vi "MultipleMissions.vi"   [LabVIEW 2014, in "LegoMindstormProjects.lvrbt"]
uses:
  LegoMindstormProjects.lvrbt
  <vilib>/NXT/Block Support/NXT_InputPort.ctl
  <vilib>/NXT/Block Support/NXT_OutputPort.ctl
  <vilib>/NXT/Subs/ColorSensorColors.ctl
  <vilib>/NXT/Dual Mode Library/Sensors/EV3_Gyro_Reset.vi
  <vilib>/NXT/NXTIO Xnodes/NXTIONodeSubVIs/NXTMoveMotors.vi
  <vilib>/NXT/Dual Mode Library/Waits/Wait_Num.vi
  <vilib>/NXT/Dual Mode Library/Sensors/EV3_Color_Color.vi
  <vilib>/NXT/NXTIO Xnodes/NXTIONodeSubVIs/NXTStopMotors.vi
  <vilib>/NXT/Dual Mode Library/Waits/Wait_EV3_Angle_Greater.vi
  <vilib>/NXT/Dual Mode Library/Waits/Wait_Rotation.vi
  <vilib>/NXT/Dual Mode Library/Waits/Wait_EV3_Angle_Less.vi
  <vilib>/NXT/NXTIO Xnodes/AddressXNode/NXTIOAddress.xnode
  <vilib>/NXT/NXTIO Xnodes/NXTIOXNode/NXTIO.xnode
  <vilib>/NXT/Subs/LVHSConnector.ctl
  <vilib>/NXT/LegoClasses/BrickReference/BrickReference.lvclass
types:
  T1 = typedef "NXT_InputPort.ctl" = u32
  T2 = typedef "NXT_OutputPort.ctl" = u8
  T3 = typedef "LVHSConnector.ctl" = refnum<class "BrickReference.lvclass">
  T4 = typedef "ColorSensorColors.ctl" = enum16{"No Color", "Black", "Blue", "Green", "Yellow", "Red", "White", "Brown"}
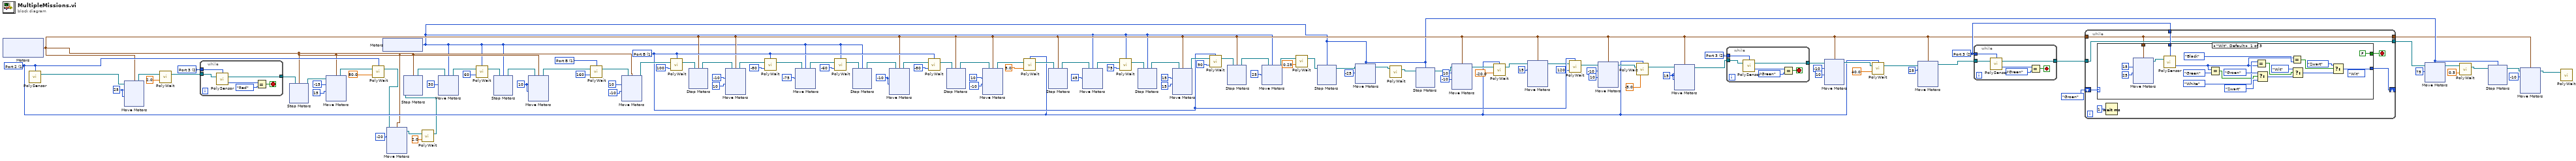
[diagram p0: block diagram]
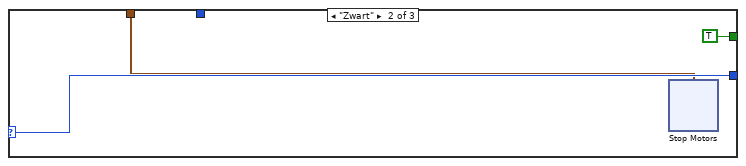
[diagram p2: hidden frame]
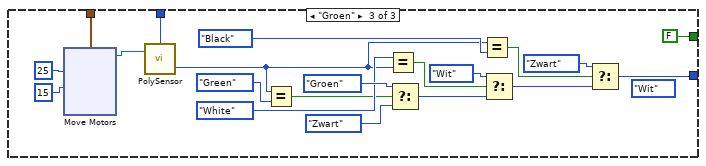
[diagram p3: hidden frame]
diagram:
  w2 = i8 -10 ("Power/Speed 1")
  w15 = i8 -20 ("Power/Speed 1")
  w19 = T1 2 items=["Port 1", "Port 2", "Port 3", "Port 4"] ("Port (Port 1)")
  w23 = i8 25 ("Power/Speed 1")
  w32 = i8 15 ("Power/Speed 1")
  w36 = T1 2 items=["Port 1", "Port 2", "Port 3", "Port 4"] ("Port (Port 1)")
  w42 = i8 15 ("Power/Speed 1")
  w59 = i8 25 ("Power/Speed 1")
  w82 = i8 -10 ("Power/Speed 1")
  w41 = T2 1 items=["Port A", "Port B", "Port C", "Port D"] ("Port (Port A)")
  w101 = T2 1 items=["Port A", "Port B", "Port C", "Port D"] ("Port (Port A)")
  w103 = i8 10 ("Power/Speed 2")
  w26 = T1 1 items=["Port 1", "Port 2", "Port 3", "Port 4"] ("Port (Port 1)")
  w116 = T1 2 items=["Port 1", "Port 2", "Port 3", "Port 4"] ("Port (Port 1)")
  n1 = xnode "Motors"() -> ("Motor"=w17:cluster{"Port":T2, "Port":T2})
  n2 = call-poly <vilib>:"PolySensor.vi"("Port (Port 1)"=w26) -> ("NXT/EV3"=w11:T3)  [unwired: 3 in]
  n3 = xnode "Move Motors"("Power/Speed 2"=w59, "Power/Speed 1"=w59, "Motors"=w17, "NXT/EV3"=w11) -> ("NXT/EV3"=w57:T3)
  n4 = call-poly <vilib>:"PolyWait.vi"("Time (1 sec)"=sgl 2.0, "NXT/EV3"=w57) -> ("NXT/EV3"=w56:T3)  [unwired: 2 in]
  n5 = while {
    tunnel: w116 -> [w122]
    tunnel: [w118] -> w115
    tunnel: w56 -> [w117]
    stop <- w119 stop-if-true
    n6 = call-poly <vilib>:"PolySensor.vi"("NXT/EV3"=w117, "Port (Port 1)"=w122) -> ("Detected Color"=w121:T4, "NXT/EV3"=w118:T3)  [unwired: 1 in]
    n7 = Equal?(x=w121, y=ColorSensorColors."Red") -> (x = y?=w119:bool)
  }
  n8 = xnode "Stop Motors"("Motors"=w17, "NXT/EV3"=w115) -> ("NXT/EV3"=w114:T3)
  n9 = xnode "Move Motors"("Power/Speed 2"=i8 15, "Power/Speed 1"=i8 -15, "Motors"=w17, "NXT/EV3"=w114) -> ("NXT/EV3"=w110:T3)
  n10 = call-poly <vilib>:"PolyWait.vi"("Degrees (180)"=sgl 80.0, "NXT/EV3"=w110, "Port (Port 1)"=w26) -> ("NXT/EV3"=w16:T3)  [unwired: 1 in]
  n11 = xnode "Motors"() -> ("Motor"=w5:T2)
  n12 = xnode "Move Motors"("Power/Speed 2"=w15, "Power/Speed 1"=w15, "Motors"=w17, "NXT/EV3"=w16) -> ("NXT/EV3"=w14:T3)
  n13 = call-poly <vilib>:"PolyWait.vi"("Time (1 sec)"=sgl 2.0, "NXT/EV3"=w14) -> ("NXT/EV3"=w12:T3)  [unwired: 2 in]
  n14 = xnode "Stop Motors"("Motors"=w17, "NXT/EV3"=w12) -> ("NXT/EV3"=w109:T3)
  n15 = xnode "Move Motors"("Power/Speed 1"=i8 30, "Motors"=w5, "NXT/EV3"=w109) -> ("NXT/EV3"=w107:T3)
  n16 = call-poly <vilib>:"PolyWait.vi"("Position Change (180)"=60, "NXT/EV3"=w107, "Port (Port A)"=w5) -> ("NXT/EV3"=w105:T3)  [unwired: 1 in]
  n17 = xnode "Stop Motors"("Motors"=w5, "NXT/EV3"=w105) -> ("NXT/EV3"=w104:T3)
  n18 = xnode "Move Motors"("Power/Speed 2"=w103, "Power/Speed 1"=w103, "Motors"=w17, "NXT/EV3"=w104) -> ("NXT/EV3"=w102:T3)
  n19 = call-poly <vilib>:"PolyWait.vi"("Position Change (180)"=160, "NXT/EV3"=w102, "Port (Port A)"=w101) -> ("NXT/EV3"=w99:T3)  [unwired: 1 in]
  n20 = xnode "Move Motors"("Power/Speed 2"=i8 -10 ("Power/Speed 1"), "Power/Speed 1"=i8 10, "Motors"=w17, "NXT/EV3"=w99) -> ("NXT/EV3"=w97:T3)
  n21 = call-poly <vilib>:"PolyWait.vi"("Position Change (180)"=100, "NXT/EV3"=w97, "Port (Port A)"=w41) -> ("NXT/EV3"=w96:T3)  [unwired: 1 in]
  n22 = xnode "Stop Motors"("Motors"=w17, "NXT/EV3"=w96) -> ("NXT/EV3"=w95:T3)
  n23 = xnode "Move Motors"("Power/Speed 2"=i8 10 ("Power/Speed 1"), "Power/Speed 1"=i8 -10, "Motors"=w17, "NXT/EV3"=w95) -> ("NXT/EV3"=w94:T3)
  n24 = call-poly <vilib>:"PolyWait.vi"("Position Change (180)"=-80, "NXT/EV3"=w94, "Port (Port A)"=w41) -> ("NXT/EV3"=w86:T3)  [unwired: 1 in]
  n25 = xnode "Move Motors"("Power/Speed 1"=i8 -75, "Motors"=w5, "NXT/EV3"=w86) -> ("NXT/EV3"=w84:T3)
  n26 = call-poly <vilib>:"PolyWait.vi"("Position Change (180)"=-60, "NXT/EV3"=w84, "Port (Port A)"=w5) -> ("NXT/EV3"=w74:T3)  [unwired: 1 in]
  n27 = xnode "Stop Motors"("Motors"=w5, "NXT/EV3"=w74) -> ("NXT/EV3"=w73:T3)
  n28 = xnode "Move Motors"("Power/Speed 2"=w82, "Power/Speed 1"=w82, "Motors"=w17, "NXT/EV3"=w73) -> ("NXT/EV3"=w88:T3)
  n29 = call-poly <vilib>:"PolyWait.vi"("Position Change (180)"=-80, "NXT/EV3"=w88, "Port (Port A)"=w41) -> ("NXT/EV3"=w81:T3)  [unwired: 1 in]
  n30 = xnode "Stop Motors"("Motors"=w17, "NXT/EV3"=w81) -> ("NXT/EV3"=w80:T3)
  n31 = xnode "Move Motors"("Power/Speed 2"=i8 -10, "Power/Speed 1"=i8 10, "Motors"=w17, "NXT/EV3"=w80) -> ("NXT/EV3"=w77:T3)
  n32 = call-poly <vilib>:"PolyWait.vi"("Degrees (180)"=sgl 5.0, "NXT/EV3"=w77, "Port (Port 1)"=w26) -> ("NXT/EV3"=w76:T3)  [unwired: 1 in]
  n33 = xnode "Stop Motors"("Motors"=w17, "NXT/EV3"=w76) -> ("NXT/EV3"=w72:T3)
  n34 = xnode "Move Motors"("Power/Speed 1"=i8 45, "Motors"=w5, "NXT/EV3"=w72) -> ("NXT/EV3"=w70:T3)
  n35 = call-poly <vilib>:"PolyWait.vi"("Position Change (180)"=75, "NXT/EV3"=w70, "Port (Port A)"=w5) -> ("NXT/EV3"=w67:T3)  [unwired: 1 in]
  n36 = xnode "Stop Motors"("Motors"=w5, "NXT/EV3"=w67) -> ("NXT/EV3"=w68:T3)
  n37 = xnode "Move Motors"("Power/Speed 2"=i8 15, "Power/Speed 1"=i8 15, "Motors"=w17, "NXT/EV3"=w68) -> ("NXT/EV3"=w64:T3)
  n38 = call-poly <vilib>:"PolyWait.vi"("Position Change (180)"=90, "NXT/EV3"=w64, "Port (Port A)"=w41) -> ("NXT/EV3"=w62:T3)  [unwired: 1 in]
  n39 = xnode "Stop Motors"("Motors"=w17, "NXT/EV3"=w62) -> ("NXT/EV3"=w61:T3)
  n40 = xnode "Move Motors"("Power/Speed 1"=i8 25, "Motors"=w5, "NXT/EV3"=w61) -> ("NXT/EV3"=w54:T3)
  n41 = call-poly <vilib>:"PolyWait.vi"("Time (1 sec)"=sgl 0.25, "NXT/EV3"=w54) -> ("NXT/EV3"=w55:T3)  [unwired: 2 in]
  n42 = xnode "Stop Motors"("Motors"=w5, "NXT/EV3"=w55) -> ("NXT/EV3"=w50:T3)
  n43 = xnode "Move Motors"("Power/Speed 1"=i8 -25, "Motors"=w5, "NXT/EV3"=w50) -> ("NXT/EV3"=w52:T3)
  n44 = call-poly <vilib>:"PolyWait.vi"("NXT/EV3"=w52) -> ("NXT/EV3"=w51:T3)  [unwired: 3 in]
  n45 = xnode "Stop Motors"("Motors"=w5, "NXT/EV3"=w51) -> ("NXT/EV3"=w48:T3)
  n46 = xnode "Move Motors"("Power/Speed 2"=i8 -10, "Power/Speed 1"=i8 10, "Motors"=w17, "NXT/EV3"=w48) -> ("NXT/EV3"=w45:T3)
  n47 = call-poly <vilib>:"PolyWait.vi"("Degrees (180)"=sgl -20.0, "NXT/EV3"=w45, "Port (Port 1)"=w26) -> ("NXT/EV3"=w43:T3)  [unwired: 1 in]
  n48 = xnode "Move Motors"("Power/Speed 2"=w42, "Power/Speed 1"=w42, "Motors"=w17, "NXT/EV3"=w43) -> ("NXT/EV3"=w40:T3)
  n49 = call-poly <vilib>:"PolyWait.vi"("Position Change (180)"=120, "NXT/EV3"=w40, "Port (Port A)"=w41) -> ("NXT/EV3"=w39:T3)  [unwired: 1 in]
  n50 = xnode "Move Motors"("Power/Speed 2"=i8 10, "Power/Speed 1"=i8 -10, "Motors"=w17, "NXT/EV3"=w39) -> ("NXT/EV3"=w35:T3)
  n51 = call-poly <vilib>:"PolyWait.vi"("Degrees (180)"=sgl -5.0, "NXT/EV3"=w35, "Port (Port 1)"=w26) -> ("NXT/EV3"=w33:T3)  [unwired: 1 in]
  n52 = xnode "Move Motors"("Power/Speed 2"=w32, "Power/Speed 1"=w32, "Motors"=w17, "NXT/EV3"=w33) -> ("NXT/EV3"=w31:T3)
  n53 = while {
    tunnel: w36 -> [w128]
    tunnel: [w124] -> w30
    tunnel: w31 -> [w123]
    stop <- w125 stop-if-true
    n54 = call-poly <vilib>:"PolySensor.vi"("NXT/EV3"=w123, "Port (Port 1)"=w128) -> ("Detected Color"=w127:T4, "NXT/EV3"=w124:T3)  [unwired: 1 in]
    n55 = Equal?(x=w127, y=ColorSensorColors."Green") -> (x = y?=w125:bool)
  }
  n56 = xnode "Move Motors"("Power/Speed 2"=i8 10, "Power/Speed 1"=i8 -10, "Motors"=w17, "NXT/EV3"=w30) -> ("NXT/EV3"=w27:T3)
  n57 = call-poly <vilib>:"PolyWait.vi"("Degrees (180)"=sgl 40.0, "NXT/EV3"=w27, "Port (Port 1)"=w26) -> ("NXT/EV3"=w24:T3)  [unwired: 1 in]
  n58 = xnode "Move Motors"("Power/Speed 2"=w23, "Power/Speed 1"=w23, "Motors"=w17, "NXT/EV3"=w24) -> ("NXT/EV3"=w22:T3)
  n59 = while {
    tunnel: w19 -> [w134]
    tunnel: [w130] -> w18
    tunnel: w22 -> [w129]
    stop <- w131 stop-if-true
    n60 = call-poly <vilib>:"PolySensor.vi"("NXT/EV3"=w129, "Port (Port 1)"=w134) -> ("Detected Color"=w133:T4, "NXT/EV3"=w130:T3)  [unwired: 1 in]
    n61 = Equal?(x=w133, y=ColorSensorColors."Green") -> (x = y?=w131:bool)
  }
  n62 = while {
    shift-right: [w139] -> _
    shift-left: enum16{"Wit", "Zwart", "Groen"}."Groen" ("Enum") -> [w140]
    tunnel: w17 -> [w135]
    tunnel: w19 -> [w137]
    tunnel: w18 -> [w136]
    tunnel: [w136] -> w10
    tunnel: [w135] -> w4
    stop <- w138 stop-if-true
    n63 = case shown="\"Wit\", Default" w140 {
      selector: w140 -> [_ w171 _]
      tunnel: [w146 w171 w182] -> w139
      tunnel: [FALSE TRUE FALSE] -> w138
      tunnel: w135 -> [w143 w170 w180]
      tunnel: w137 -> [w144 _ w179]
      frame "Wit", Default {
        (unwired) enum16{"Wit", "Zwart", "Groen"}."Wit" ("Enum")
        n64 = xnode "Move Motors"("Power/Speed 2"=i8 25, "Power/Speed 1"=i8 15 ("Power/Speed 2"), "Motors"=w143) -> ("NXT/EV3"=w148:T3)  [unwired: 1 in]
        n65 = call-poly <vilib>:"PolySensor.vi"("NXT/EV3"=w148, "Port (Port 1)"=w144) -> ("Detected Color"=w153:T4)  [unwired: 1 in, 1 out]
        n66 = Equal?(x=w153, y=ColorSensorColors."Green") -> (x = y?=w150:bool)
        n67 = Equal?(x=ColorSensorColors."White" ("y"), y=w153) -> (x = y?=w152:bool)
        n68 = Select(t=enum16{"Wit", "Zwart", "Groen"}."Groen" ("Enum"), s=w150, f=enum16{"Wit", "Zwart", "Groen"}."Zwart" ("Enum")) -> (s? t:f=w151:enum16{"Wit", "Zwart", "Groen"})
        n69 = Equal?(x=w153, y=ColorSensorColors."Black") -> (x = y?=w154:bool)
        n70 = Select(t=enum16{"Wit", "Zwart", "Groen"}."Wit" ("Enum"), s=w152, f=w151) -> (s? t:f=w155:enum16{"Wit", "Zwart", "Groen"})
        n71 = Select(t=enum16{"Wit", "Zwart", "Groen"}."Zwart" ("Enum"), s=w154, f=w155) -> (s? t:f=w146:enum16{"Wit", "Zwart", "Groen"})
      }
      frame "Zwart" {
        n72 = xnode "Stop Motors"("Motors"=w170) -> ()  [unwired: 1 in, 1 out]
      }
      frame "Groen" {
        (unwired) enum16{"Wit", "Zwart", "Groen"}."Wit" ("Enum")
        n73 = xnode "Move Motors"("Power/Speed 2"=i8 15, "Power/Speed 1"=i8 25 ("Power/Speed 2"), "Motors"=w180) -> ("NXT/EV3"=w184:T3)  [unwired: 1 in]
        n74 = call-poly <vilib>:"PolySensor.vi"("NXT/EV3"=w184, "Port (Port 1)"=w179) -> ("Detected Color"=w189:T4)  [unwired: 1 in, 1 out]
        n75 = Equal?(x=w189, y=ColorSensorColors."Green") -> (x = y?=w186:bool)
        n76 = Equal?(x=ColorSensorColors."White" ("y"), y=w189) -> (x = y?=w188:bool)
        n77 = Select(t=enum16{"Wit", "Zwart", "Groen"}."Groen" ("Enum"), s=w186, f=enum16{"Wit", "Zwart", "Groen"}."Zwart" ("Enum")) -> (s? t:f=w187:enum16{"Wit", "Zwart", "Groen"})
        n78 = Equal?(x=w189, y=ColorSensorColors."Black") -> (x = y?=w190:bool)
        n79 = Select(t=enum16{"Wit", "Zwart", "Groen"}."Wit" ("Enum"), s=w188, f=w187) -> (s? t:f=w191:enum16{"Wit", "Zwart", "Groen"})
        n80 = Select(t=enum16{"Wit", "Zwart", "Groen"}."Zwart" ("Enum"), s=w190, f=w191) -> (s? t:f=w182:enum16{"Wit", "Zwart", "Groen"})
      }
    }
    n81 = Wait (ms)(milliseconds to wait=u32 1) -> ()  [unwired: 1 out]
  }
  n82 = xnode "Move Motors"("Power/Speed 1"=i8 75, "Motors"=w5, "NXT/EV3"=w10) -> ("NXT/EV3"=w8:T3)
  n83 = call-poly <vilib>:"PolyWait.vi"("Time (1 sec)"=sgl 0.5, "NXT/EV3"=w8) -> ("NXT/EV3"=w6:T3)  [unwired: 2 in]
  n84 = xnode "Stop Motors"("Motors"=w5, "NXT/EV3"=w6) -> ("NXT/EV3"=w3:T3)
  n85 = xnode "Move Motors"("Power/Speed 2"=w2, "Power/Speed 1"=w2, "Motors"=w4, "NXT/EV3"=w3) -> ("NXT/EV3"=w1:T3)
  n86 = call-poly <vilib>:"PolyWait.vi"("NXT/EV3"=w1) -> ()  [unwired: 3 in, 1 out]
